vi "SMTP Email Get Next Line.vi"(3 "last chunk":bool, 5 "string":string) -> (0 "found eoln":bool, 1 "after eoln":string, 2 "before eoln":string)   [LabVIEW 2012, in "NewNI_SMTPEmail.lvlib"]
uses:
  NewNI_SMTPEmail.lvlib
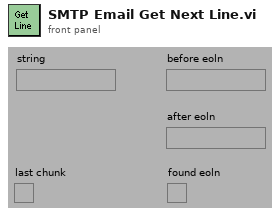
[diagram p1: front panel]
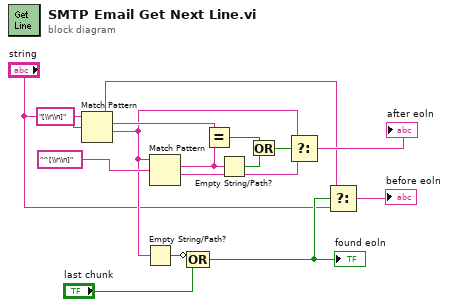
[diagram p0: block diagram]
diagram:
  n1 = Match Pattern(string="string", regular expression="[\\r\\n]") -> (before substring=w2:string, match substring=w14:string, after substring=w7:string)  [unwired: 2 out]
  n2 = Empty String/Path?(string/path=w7) -> (empty?=w6:bool)
  n3 = Match Pattern(string=w7, regular expression="^[\\r\\n]") -> (match substring=w13:string, after substring=w8:string)  [unwired: 3 out]
  n4 = Compound Arithmetic op=OR(invert w6, "last chunk") -> (w4:bool)
  "found eoln" <- w4
  n5 = Equal?(x=w14, y=w13) -> (x = y?=w12:bool)
  n6 = Empty String/Path?(string/path=w13) -> (empty?=w11:bool)
  n7 = Or(x=w12, y=w11) -> (x .or. y?=w10:bool)
  n8 = Select(t=w7, s=w10, f=w8) -> (s? t:f=→"after eoln":string)
  n9 = Select(t=w2, s=w4, f="string") -> (s? t:f=→"before eoln":string)
